vi "data_download_shuzu.vi"(8 "文件路径（使用对话框）":path, 10 "数组":dbl[](array[numeric])) -> ()   [LabVIEW 2020]
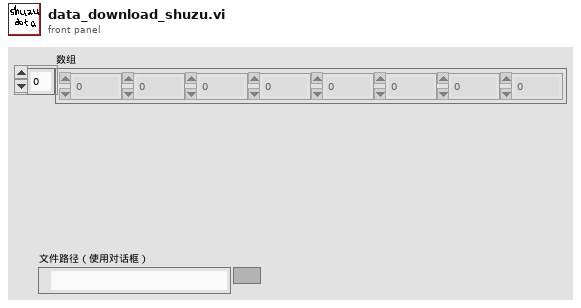
[diagram p1: front panel]
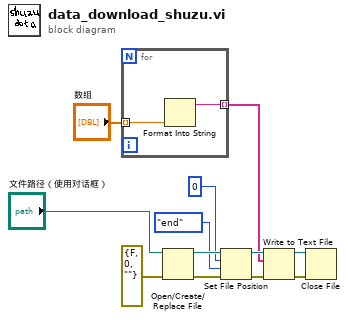
[diagram p0: block diagram]
diagram:
  n1 = for {
    tunnel: "数组" -> [w14] mode=indexing
    tunnel: [w13] -> w5 mode=indexing
    n2 = Format Into String(w14) -> (resulting string=w13:string)  [unwired: 3 in, 1 out]
  }
  n3 = Open/Create/Replace File(file path (use dialog)="文件路径（使用对话框）", error in=errorcluster {"status"=FALSE, "code"=0, "source"=""} ("错误输入")) -> (refnum out=w9:refnum<file>, error out=w11:errorcluster)  [unwired: 4 in, 1 out]
  n4 = Set File Position(offset (in bytes) (0)=i64 0 ("偏移量（字节）（0）"), refnum=w9, from (0:start)=enum16{"start", "end", "current"}."end" ("自（0:起始）"), error in=w11) -> (refnum out=w8:refnum<file>, error out=w10:errorcluster)
  n5 = Write to Text File(file (use dialog)=w8, text=w5, error in=w10) -> (refnum out=w4:refnum<file>, error out=w3:errorcluster)  [unwired: 1 in, 1 out]
  n6 = Close File(refnum=w4, error in=w3) -> ()  [unwired: 2 out]
